vi "parms.vi"(1 "dimensions":i64[](array[numeric])=[1399090569999999999, -1], 2 "values":cluster{"banana":i16, "foo":string}[](array[cluster])=[{"banana"=42, "foo"="bar"}], 3 "label":string="parms") -> (0 "JSON string":string="{\"label\":\"parms\",\"values\":[{\"banana\":42,\"foo\":\"bar\\nbar\"}],\"dimensions\":[1399090569999999999,-1]}")   [LabVIEW 2014]
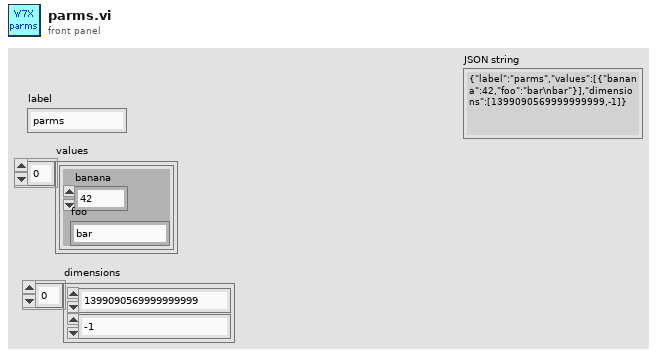
[diagram p1: front panel]
types:
  T1 = cluster{"label":string, "values":cluster{"banana":i16, "foo":string}[], "dimensions":i64[]}
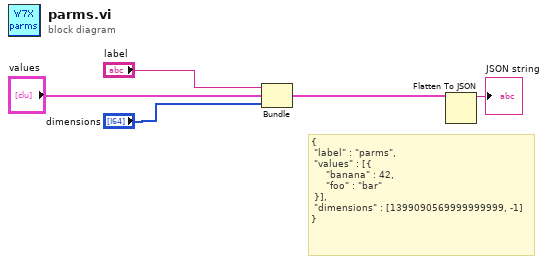
[diagram p0: block diagram]
diagram:
  # "{\n \"label\" : \"parms\",\n \"values\" : [{\n     \"banana\" : 42,\n     \"foo\" : \"bar\"\n }],\n \"dimensions\" : [1399090569999999999, -1]\n}"
  n1 = Bundle("label"="label", "values"="values", "dimensions"="dimensions") -> (w2:T1)  [unwired: 1 in]
  n2 = Flatten To JSON(anything=w2) -> (JSON string=→"JSON string":string)  [unwired: 2 in, 1 out]
